vi "SVMM plugin framework.vi"() -> ()   [LabVIEW 2022 SP3]
doc: "Model Thread API Tester."
uses:
  Abstract View/Abstract View.lvlibp/Abstract View.lvclass
  Libraries/Model Thread/Model Thread.lvlib
panel:
  out "SVMM plug-in framework":string
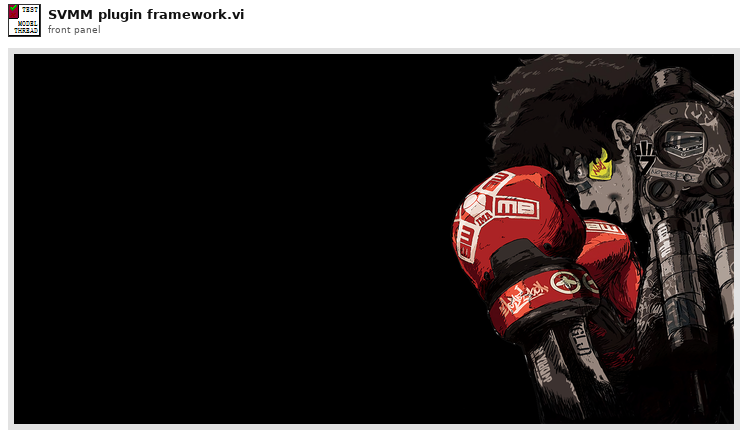
[diagram p1: front panel]
types:
  T1 = enum32{"Invalid", "Standard", "Closed", "Hidden", "Minimized", "Maximized"}
  T2 = typedef "Model Thread.lvlib/Broadcast Events--cluster.ctl" = cluster{"Module Did Init":refnum<user-event>, "Status Updated":refnum<user-event>, "Error Reported":refnum<user-event>, "Module Did Stop":refnum<user-event>, "Update Module Execution Status":refnum<user-event>, "data change":refnum<user-event>}
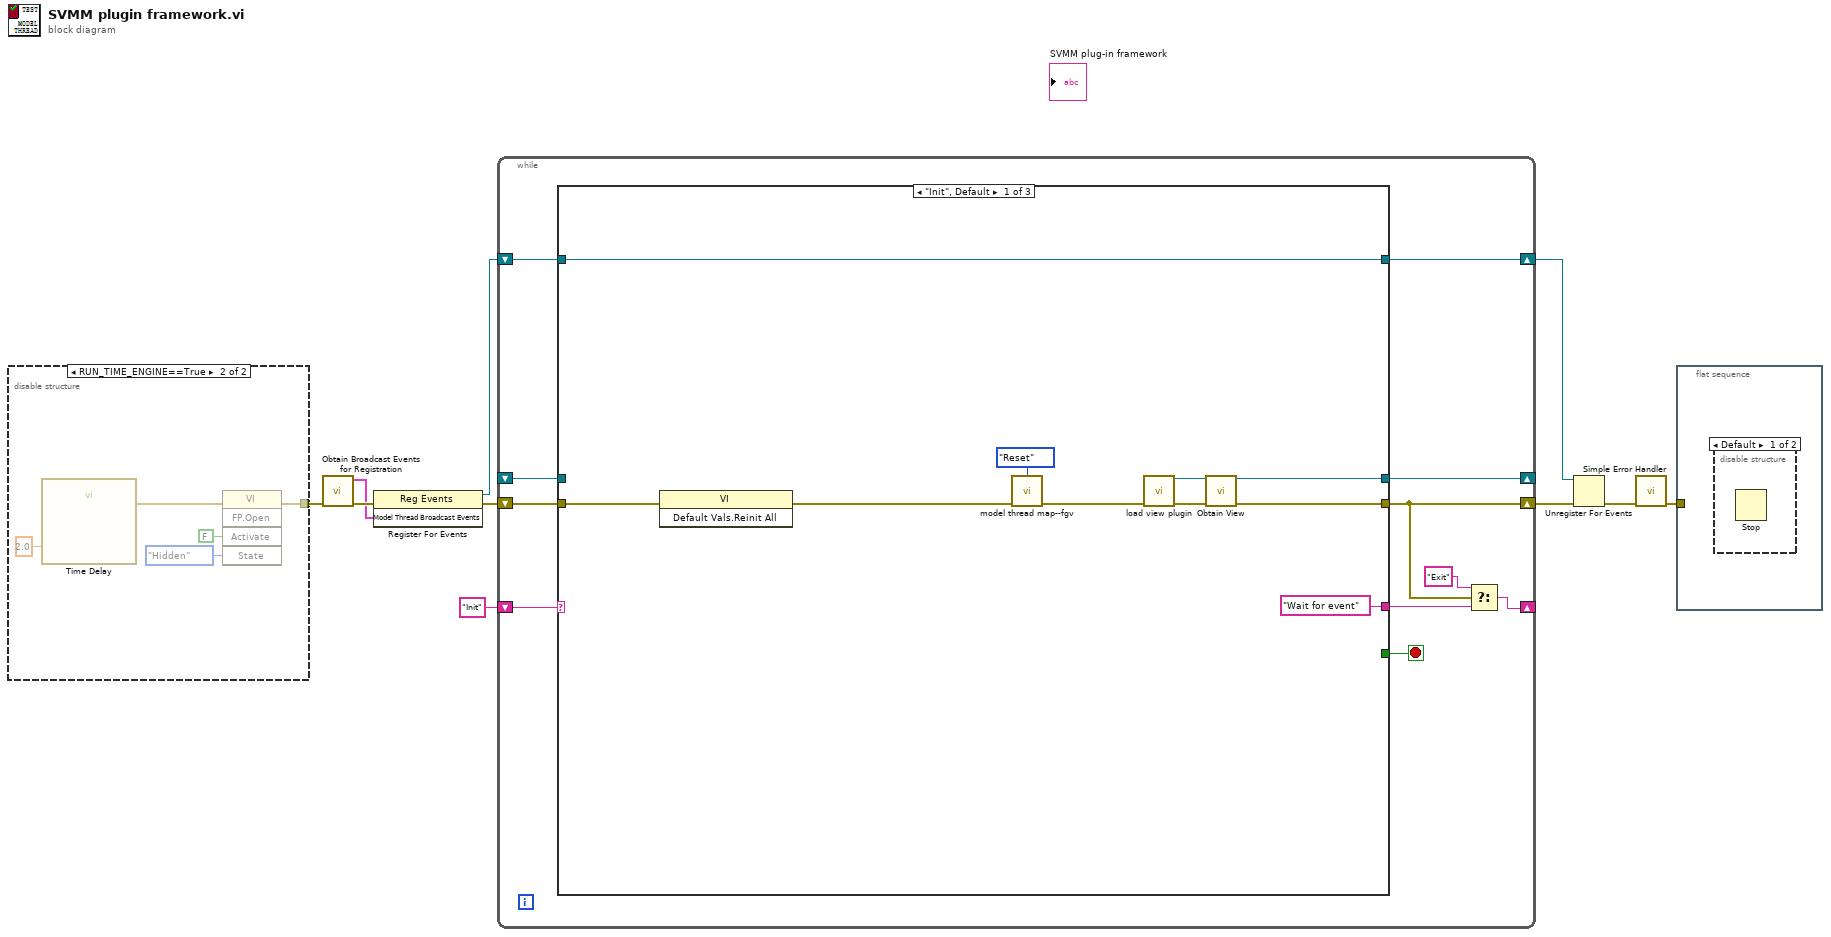
[diagram p0: block diagram]
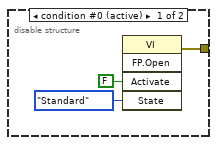
[diagram p2: hidden frame]
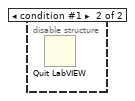
[diagram p3: hidden frame]
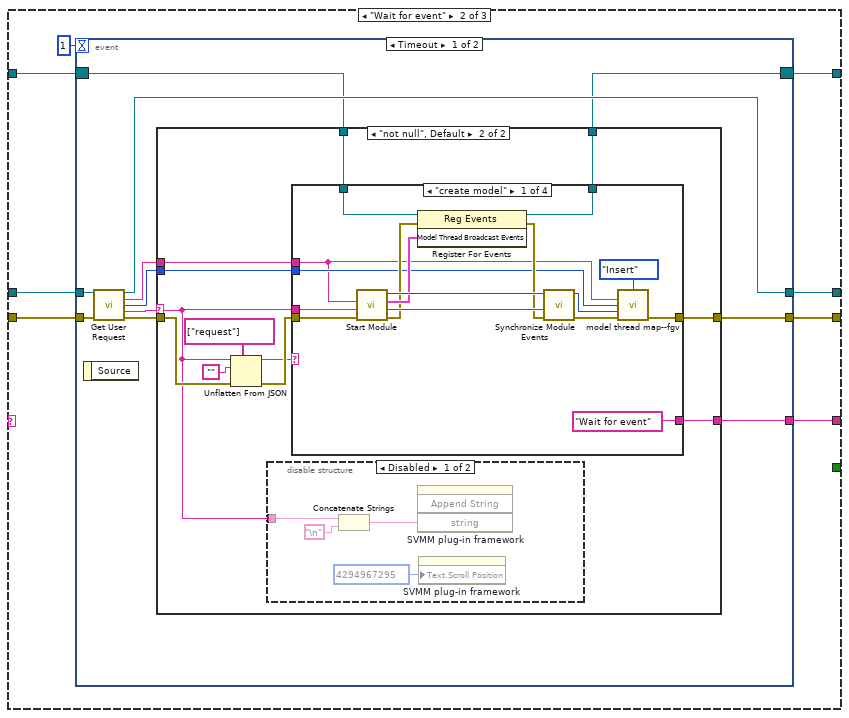
[diagram p4: hidden frame]
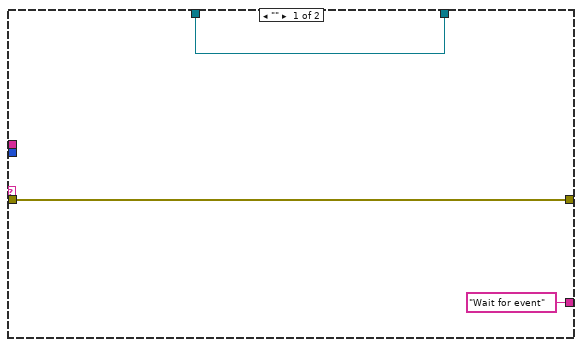
[diagram p5: hidden frame]
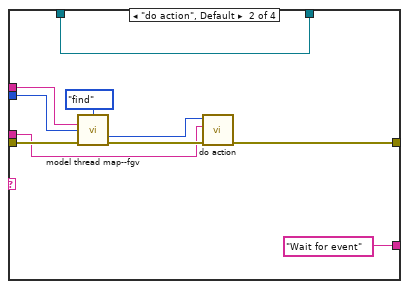
[diagram p7: hidden frame]
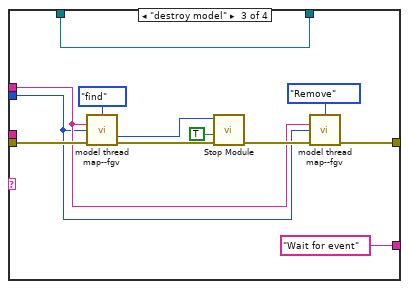
[diagram p8: hidden frame]
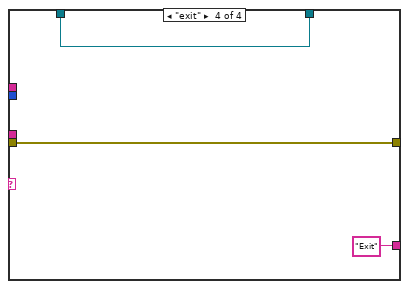
[diagram p9: hidden frame]
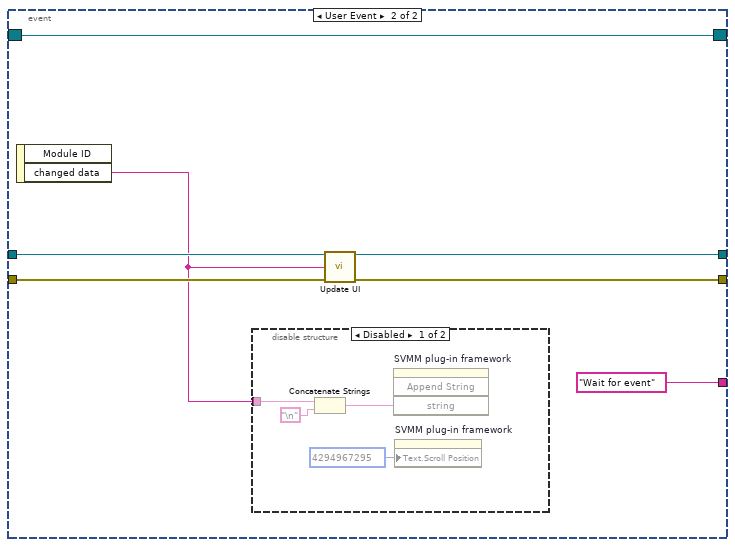
[diagram p10: hidden frame]
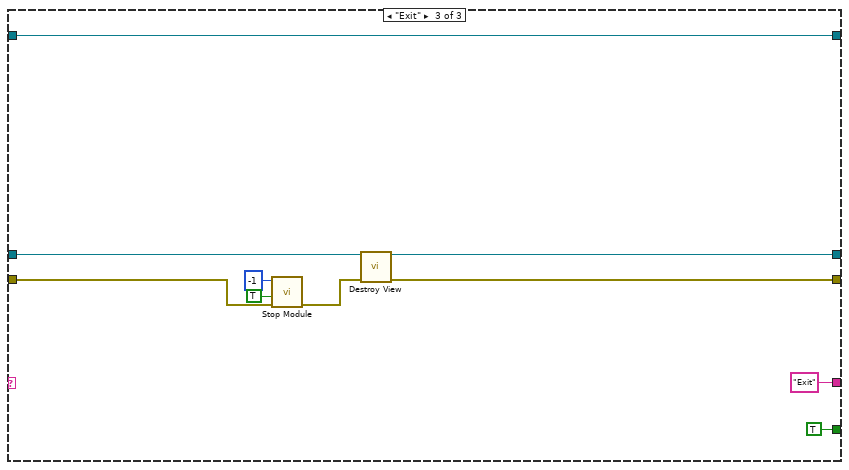
[diagram p12: hidden frame]
diagram:
  n1 = disable-structure shown="RUN_TIME_ENGINE==True" {
    disable-tunnel: [w13 w18] -> w1
    frame condition #0 (active) {
      n2 = invoke class="VI" method="FP.Open"("Activate"=FALSE ("Activate?"), "State"=T1."Standard") -> (error out=w13:errorcluster)  [unwired: 3 in, 4 out]
    }
    frame condition #1 {
      n3 = call "Time Delay"("Delay Time (s)"=2.0) -> ("error out"=w14:errorcluster)  [unwired: 10 in]
      n4 = invoke class="VI" method="FP.Open"(error in=w14, "Activate"=FALSE ("Activate?"), "State"=T1."Hidden") -> (error out=w18:errorcluster)  [unwired: 2 in, 4 out]
    }
  }
  n5 = call "Obtain Broadcast Events for Registration.vi"("error in"=w1) -> ("error out"=w9:errorcluster, "Model Thread Broadcast Events"=w7:T2)  [unwired: 8 in, 1 out]
  n6 = register-events(error in=w9, w7) -> (reference out=w6:refnum<event-registration>, error out=w8:errorcluster)  [unwired: 1 in]
  n7 = while {
    shift-right: [w20] -> _
    shift-left: "Init" -> [w28]
    shift-right: [w27] -> _
    shift-left: _ -> [w26]
    shift-right: [w24] -> w5
    shift-left: w6 -> [w25]
    shift-right: [w23] -> w3
    shift-left: w8 -> [w29]
    stop <- w19 stop-if-true
    n8 = case shown="\"Init\", Default" w28 {
      tunnel: w29 -> [w31 w47 w133]
      tunnel: [w39 w44 w138] -> w23
      tunnel: [w38 w43 w137] -> w27
      tunnel: ["Wait for event" w40 "Exit"] -> w22
      tunnel: w26 -> [_ w45 w136]
      tunnel: w25 -> [w36 w42 w139]
      tunnel: [w36 w41 w139] -> w24
      tunnel: [_ _ TRUE] -> w19
      frame "Init", Default {
        n9 = invoke class="VI" method="Default Vals.Reinit All"(error in=w31) -> (error out=w30:errorcluster)  [unwired: 2 in, 2 out]
        n10 = call "model thread map--fgv.vi"("operation"=enum16{"Reset", "Insert", "Remove", "find"}."Reset", "error in (no error)"=w30) -> ("error out"=w35:errorcluster)  [unwired: 9 in, 4 out]
        n11 = call "load view plugin.vi"("error in (no error)"=w35) -> ("view plugin"=w33:refnum<class "Abstract View.lvclass">, "error out"=w34:errorcluster)  [unwired: 13 in]
        n12 = call-dynamic "Obtain View.vi"("Abstract View in"=w33, "error in (no error)"=w34) -> ("Abstract View out"=w38:refnum<class "Abstract View.lvclass">, "error out"=w39:errorcluster)  [unwired: 12 in]
      }
      frame "Wait for event" {
        n13 = event shown="[0] Timeout" {
          selector: w42 -> [w54 w120]
          dyn-events: [w53 w120] -> w41
          timeout: 1 -> [_ _]
          tunnel: w47 -> [w58 w125]
          tunnel: w45 -> [w57 w123]
          tunnel: [w55 w124] -> w44
          tunnel: [w56 w122] -> w43
          tunnel: [w52 "Wait for event"] -> w40
          event Timeout {
            n14 = event-data() -> ()  [unwired: 1 in, 1 out]
            n15 = call-dynamic "Get User Request.vi"("Abstract View in"=w57, "error in (no error)"=w58) -> ("Abstract View out"=w56:refnum<class "Abstract View.lvclass">, "Model Name"=w51:string, "Model Number"=w50:i32, "Request"=w48:string, "error out"=w49:errorcluster)  [unwired: 9 in]
            n16 = case shown="\"not null\", Default" w48 {
              selector: w48 -> [_ w62]
              tunnel: [w61 w73] -> w55
              tunnel: w54 -> [w59 w72]
              tunnel: [w59 w71] -> w53
              tunnel: ["Wait for event" w70] -> w52
              tunnel: w49 -> [w61 w65]
              tunnel: w51 -> [_ w69]
              tunnel: w50 -> [_ w68]
              frame "" {
              }
              frame "not null", Default {
                n17 = Unflatten From JSON(path=string[] ["request"], JSON string=w62, type and defaults="", error in (no error)=w65) -> (value=w63:string, error out=w64:errorcluster)  [unwired: 3 in]
                n18 = disable-structure shown="Disabled" {
                  disable-tunnel: w62 -> [w74 _]
                  frame Disabled {
                    n19 = Concatenate Strings(w74, "\n") -> (w77:string)
                    n20 = invoke on="SVMM plug-in framework" class="Str" method="Append String"("string"=w77) -> ()  [unwired: 3 in, 4 out]
                    n21 = property on="SVMM plug-in framework" class="Str"("Text.Scroll Position"=u32 4294967295) -> ()  [unwired: 2 in, 2 out]
                  }
                  frame Enabled {
                  }
                }
                n22 = case shown="\"create model\"" w63 {
                  tunnel: w64 -> [w88 w102 w114 w118]
                  tunnel: w72 -> [w87 w103 w115 w116]
                  tunnel: [w86 w103 w115 w116] -> w71
                  tunnel: [w83 w98 w107 w118] -> w73
                  tunnel: w69 -> [w81 w101 w105 _]
                  tunnel: w68 -> [w82 w100 w104 _]
                  tunnel: w62 -> [w80 w96 _ _]
                  tunnel: ["Wait for event" "Wait for event" "Wait for event" "Exit"] -> w70
                  frame "create model" {
                    n23 = call "Start Module.vi"("error in"=w88, "init information"=w80, "model name"=w81) -> ("error out"=w90:errorcluster, "Wait for Event Sync?"=w91:bool, "Model Thread Broadcast Events"=w92:T2, "Module ID"=w93:i32)  [unwired: 5 in]
                    n24 = register-events(reference=w87, error in=w90, w92) -> (reference out=w86:refnum<event-registration>, error out=w89:errorcluster)
                    n25 = call "Synchronize Module Events.vi"("error in"=w89, "Wait for Event Sync?"=w91, "Module ID in"=w93) -> ("error out"=w85:errorcluster, "Module ID out"=w84:i32)  [unwired: 7 in]
                    n26 = call "model thread map--fgv.vi"("operation"=enum16{"Reset", "Insert", "Remove", "find"}."Insert", "model name in"=w81, "model number in"=w82, "thread number In"=w84, "error in (no error)"=w85) -> ("error out"=w83:errorcluster)  [unwired: 6 in, 4 out]
                  }
                  frame "do action", Default {
                    n27 = call "model thread map--fgv.vi"("operation"=enum16{"Reset", "Insert", "Remove", "find"}."find", "model name in"=w101, "model number in"=w100, "error in (no error)"=w102) -> ("thread number out"=w97:i32, "error out"=w99:errorcluster)  [unwired: 7 in, 3 out]
                    n28 = call "do action.vi"("error in"=w99, "request"=w96, "Module ID"=w97) -> ("error out"=w98:errorcluster)  [unwired: 8 in]
                  }
                  frame "destroy model" {
                    n29 = call "model thread map--fgv.vi"("operation"=enum16{"Reset", "Insert", "Remove", "find"}."find", "model name in"=w105, "model number in"=w104, "error in (no error)"=w114) -> ("thread number out"=w112:i32, "error out"=w113:errorcluster)  [unwired: 7 in, 3 out]
                    n30 = call "Stop Module.vi"("error in"=w113, "Wait for Module to stop? (F)"=TRUE, "Module ID"=w112) -> ("error out"=w108:errorcluster)  [unwired: 8 in]
                    n31 = call "model thread map--fgv.vi"("operation"=enum16{"Reset", "Insert", "Remove", "find"}."Remove", "model name in"=w105, "model number in"=w104, "error in (no error)"=w108) -> ("error out"=w107:errorcluster)  [unwired: 7 in, 4 out]
                  }
                  frame "exit" {
                  }
                }
              }
            }
          }
          event User Event {
            n32 = event-data() -> ("changed data"=w119:string)  [unwired: 1 in, 1 out]
            n33 = disable-structure shown="Disabled" {
              disable-tunnel: w119 -> [w126 _]
              frame Disabled {
                n34 = Concatenate Strings(w126, "\n") -> (w129:string)
                n35 = invoke on="SVMM plug-in framework" class="Str" method="Append String"("string"=w129) -> ()  [unwired: 3 in, 4 out]
                n36 = property on="SVMM plug-in framework" class="Str"("Text.Scroll Position"=u32 4294967295) -> ()  [unwired: 2 in, 2 out]
              }
              frame Enabled {
              }
            }
            n37 = call-dynamic "Update UI.vi"("Abstract View in"=w123, "changed data"=w119, "error in (no error)"=w125) -> ("Abstract View out"=w122:refnum<class "Abstract View.lvclass">, "error out"=w124:errorcluster)  [unwired: 11 in]
          }
        }
      }
      frame "Exit" {
        n38 = call "Stop Module.vi"("error in"=w133, "Wait for Module to stop? (F)"=TRUE, "Module ID"=-1) -> ("error out"=w132:errorcluster)  [unwired: 8 in]
        n39 = call-dynamic "Destroy View.vi"("Abstract View in"=w136, "error in (no error)"=w132) -> ("Abstract View out"=w137:refnum<class "Abstract View.lvclass">, "error out"=w138:errorcluster)  [unwired: 12 in]
      }
    }
    n40 = Select(t="Exit", s=w23, f=w22) -> (s? t:f=w20:string)
  }
  n41 = Unregister For Events(event registration refnum=w5, error in=w3) -> (error out=w4:errorcluster)
  n42 = call <vilib>:"Simple Error Handler.vi"("error in (no error)"=w4) -> ("error out"=w2:errorcluster)  [unwired: 4 in, 4 out]
  n43 = flat-sequence {
    tunnel: w2 -> [_]
    frame #0 {
      n44 = disable-structure shown="Default" {
        frame condition #0 (active) {
          n45 = Stop() -> ()  [unwired: 1 in]
        }
        frame condition #1 {
          n46 = Quit LabVIEW() -> ()  [unwired: 1 in]
        }
      }
    }
  }
